vi "Autoscroll.vi"(8 "error in (no error)":errorcluster, 11 "String Control Sink in":refnum<class "String Control Sink.lvclass">) -> (0 "error out":errorcluster, 3 "String Control Sink out":refnum<class "String Control Sink.lvclass">)   [LabVIEW 2017, in "String Control Sink.lvclass"]
uses:
  String Control Sink.lvclass
  String Control Sink.lvclass/String Control Sink.ctl
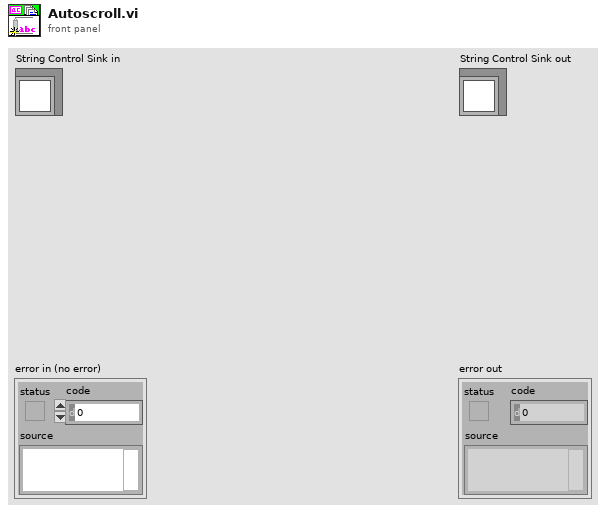
[diagram p1: front panel]
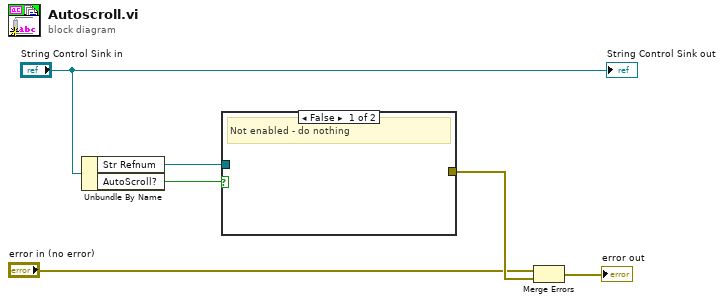
[diagram p0: block diagram]
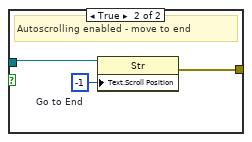
[diagram p2: hidden frame]
diagram:
  n1 = Unbundle By Name("String Control Sink in") -> ("Str Refnum"=w4:refnum<vi>, "AutoScroll?"=w5:bool)
  n2 = case shown="False" w5 {
    tunnel: w4 -> [_ w9]
    tunnel: [_ w7] -> w3
    frame False {
      # "Not enabled - do nothing"
    }
    frame True {
      w8 = -1  # Go to End
      # "Autoscrolling enabled - move to end"
      n3 = property class="Str"(reference=w9, "Text.Scroll Position"=w8) -> (error out=w7:errorcluster)  [unwired: 1 in, 1 out]
    }
  }
  n4 = Merge Errors("error in (no error)", w3) -> (→"error out":errorcluster)
  "String Control Sink out" <- "String Control Sink in"
